vi "mode switching exmple.vi"() -> ()   [LabVIEW 2020]
uses:
  SEC Software V3.0/SEC code V3.0.1/Drivers and Aux files/IVIUM/IVIUM_remdriver.lvlib
panel:
  in  "Default\nCurrent range":T1(ring)=enum."100 uA"
  in  "Default Filter":T2(ring)=enum."10 kHz"
  in  "Set Stability":T3(ring)=enum."Standard"
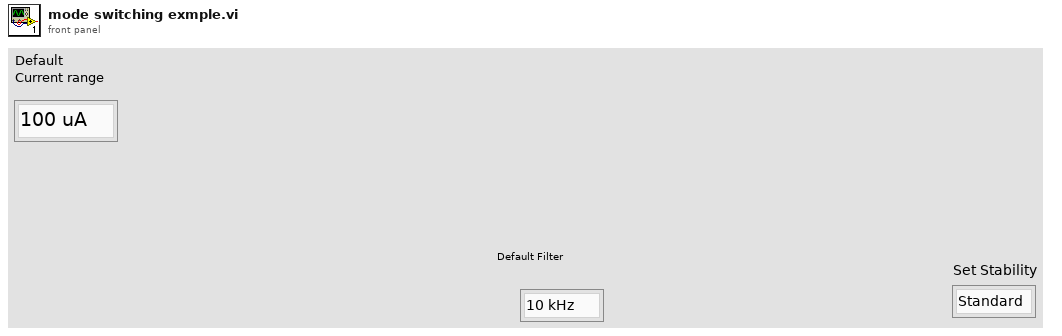
[diagram p1: front panel]
types:
  T1 = enum16{"10 A", "1 A", "100 mA", "10 mA", "1 mA", "100 uA", "10 uA", "1 uA", "100 nA", "10 nA", "1 nA", "100 pA", "10 pA", "1 pA"}
  T2 = enum16{"1 MHz", "100 kHz", "10 kHz", "1 kHz", "10 Hz"}
  T3 = enum16{"High Speed", "Standard", "High Stability"}
  T4 = cluster{"Current array":dbl[], "Potential array":dbl[], "Status":string, "Serial No":string, "Current":dbl, "Default\n potential":dbl, "I overload":bool, "Cell on":bool, "E overload":bool, "Cell of button pressed":bool, "Aninput1 overload":bool, "Stop \npotential":dbl, "Start \npotential":dbl, "Increment":dbl, "Spectrum":dbl[][], "Path":path, "File Name":string, "Sample rate":dbl, "V2 time":dbl, "V off time":dbl, "V 2":dbl, "V 1":dbl, "V1 time":dbl, "Time array":dbl[], "Integration time":i32, "Continous strobe delay":i32, "Time elapsed ":i32, "Start time":i32}
  T5 = enum16{"off", "EStat4EL", "EStat2EL", "EStatDummy1", "EStatDummy2", "EStatDummy3", "EStatDummy4", "IStat4EL", "IStat2EL", "IStatDummy", "BiStat4EL", "BiStat2EL"}
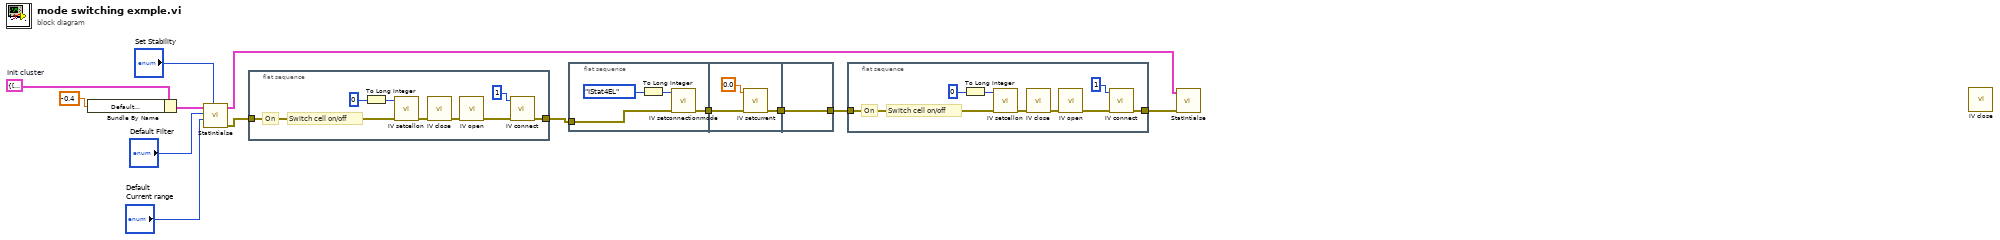
[diagram p0: block diagram]
diagram:
  w13 = T4 {"Current array"=[], "Potential array"=[], "Status"="", "Serial No"="", "Current"=0.0, "Default\n potential"=0.0, "I overload"=FALSE, "Cell on"=FALSE, "E overload"=FALSE, "Cell of button pressed"=FALSE, "Aninput1 overload"=FALSE, "Stop \npotential"=0.0, "Start \npotential"=0.0, "Increment"=0.0, "Spectrum"=[], "Path"=path "", "File Name"="", "Sample rate"=0.0, "V2 time"=0.0, "V off time"=0.0, "V 2"=0.0, "V 1"=0.0, "V1 time"=0.0, "Time array"=[], "Integration time"=0, "Continous strobe delay"=0, "Time elapsed "=0, "Start time"=0}  # Init cluster
  n1 = Bundle By Name(cluster=w13, "Default\n potential"=-0.4 ("Default\n potential")) -> (w11:T4)
  n2 = call "StatIntialse.vi"("Set Stability"="Set Stability", "Default\nCurrent range"="Default\nCurrent range", "Default\n Filter"="Default Filter", "Cluster in"=w11) -> ("error out"=w3:errorcluster, "Cluster out"=w1:T4)  [unwired: 6 in]
  n3 = flat-sequence {
    tunnel: [w14] -> _
    tunnel: w3 -> [w16]
    tunnel: [w14] -> w2
    frame #0 {
      # "On"
      # "Switch cell on/off"
      n4 = To Long Integer(number=0) -> (32bit integer=w18:i32)
      n5 = call "IV setcellon.vi"("error in (no error)"=w16, "cellon"=w18) -> ("error out"=w15:errorcluster)  [unwired: 7 in, 2 out]
      n6 = call "IV close.vi"("error in (no error)"=w15) -> ("error out"=w20:errorcluster)  [unwired: 9 in, 1 out]
      n7 = call "IV open.vi"("error in (no error)"=w20) -> ("error out"=w19:errorcluster)  [unwired: 9 in, 1 out]
      n8 = call "IV connect.vi"("error in (no error)"=w19, "devconnect"=1) -> ("error out"=w14:errorcluster)  [unwired: 7 in, 2 out]
    }
  }
  n9 = flat-sequence {
    tunnel: w2 -> [w25]
    tunnel: [w24] -> w10
    tunnel: w10 -> [w28]
    tunnel: [w27] -> w9
    tunnel: [w29] -> w6
    tunnel: w9 -> [w29]
    frame #0 {
      n10 = To Long Integer(number=T5."IStat4EL" ("Configuration")) -> (32bit integer=w23:i32)
      n11 = call "IV setconnectionmode.vi"("error in (no error)"=w25, "value"=w23) -> ("error out"=w24:errorcluster)  [unwired: 7 in, 2 out]
    }
    frame #1 {
      n12 = call "IV setcurrent.vi"("error in (no error)"=w28, "value"=0.0) -> ("error out"=w27:errorcluster)  [unwired: 7 in, 2 out]
    }
    frame #2 {
    }
  }
  n13 = flat-sequence {
    tunnel: [w34] -> w8
    tunnel: w6 -> [w31]
    frame #0 {
      # "On"
      # "Switch cell on/off"
      n14 = To Long Integer(number=0) -> (32bit integer=w33:i32)
      n15 = call "IV setcellon.vi"("error in (no error)"=w31, "cellon"=w33) -> ("error out"=w30:errorcluster)  [unwired: 7 in, 2 out]
      n16 = call "IV close.vi"("error in (no error)"=w30) -> ("error out"=w36:errorcluster)  [unwired: 9 in, 1 out]
      n17 = call "IV open.vi"("error in (no error)"=w36) -> ("error out"=w35:errorcluster)  [unwired: 9 in, 1 out]
      n18 = call "IV connect.vi"("error in (no error)"=w35, "devconnect"=1) -> ("error out"=w34:errorcluster)  [unwired: 7 in, 2 out]
    }
  }
  n19 = call "StatIntialse.vi"("error in (no error)"=w8, "Cluster in"=w1) -> ()  [unwired: 8 in, 2 out]
  n20 = call "IV close.vi"() -> ()  [unwired: 10 in, 2 out]
